vi "Two Force Sensors V3.vi"(8 "error out":errorcluster, 9 "Analog Input Pin 2":u8, 10 "Analog Input Pin1":u8, 11 "Arduino Resource":T1={"VISA resource"="", "Board Type"=enum."Uno", "Connection Type"=enum."USB / Serial", "Bytes Per Packet (15)"=15}) -> (0 "error out 2":errorcluster, 2 "Average Force":dbl(graph), 3 "Arduino Resource 2":T1={"VISA resource"="", "Board Type"=enum."Uno", "Connection Type"=enum."USB / Serial", "Bytes Per Packet (15)"=15})   [LabVIEW 2013]
uses:
  <vilib>/LabVIEW Interface for Arduino/Type Defs/Arduino Resource.ctl
  <vilib>/LabVIEW Interface for Arduino/Type Defs/Board Type.ctl
  <vilib>/Analysis/baseanly.llb/Mean (DBL).vi
  <vilib>/LabVIEW Interface for Arduino/LabVIEW Interface for Arduino.lvlib
  <vilib>/Analysis/NI_AALBase.lvlib
panel:
  out "Average Force":dbl
  out "Force2 Average":dbl format="%0.2f"
  out "Force1 Average":dbl format="%0.2f"
  out "Force 2":dbl(graph)
  out "Voltage2":dbl(graph)
  out "Force":dbl(graph)
  in  "Array":dbl[](array[numeric])
  in  "Stop":bool
  out "Volatge":dbl(graph)
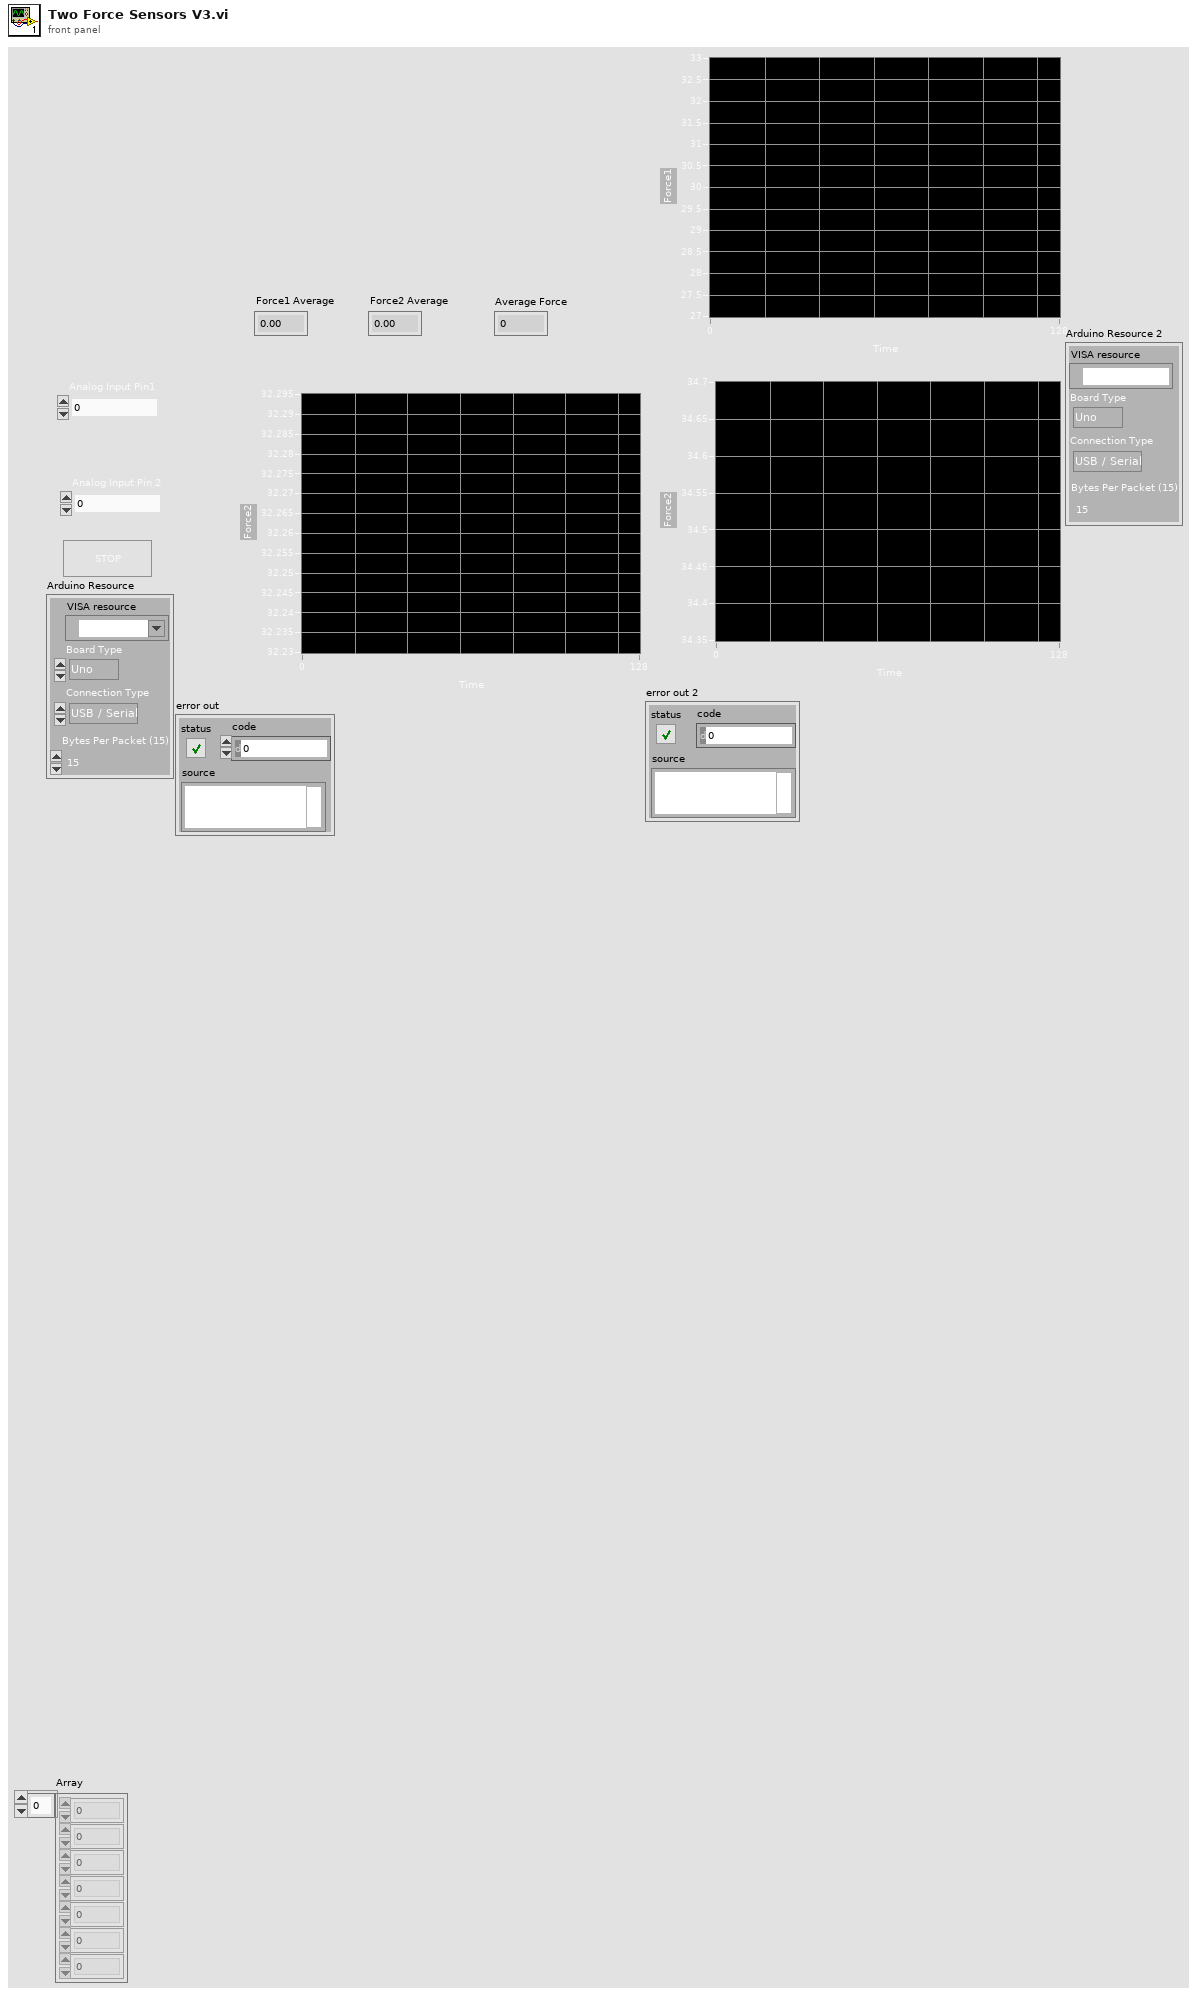
[diagram p1: front panel]
types:
  T1 = typedef "LabVIEW Interface for Arduino.lvlib/Arduino Resource.ctl" = cluster{"VISA resource":refnum<visa-resource-name>, "Board Type":T2, "Connection Type":enum8{"USB / Serial"}, "Bytes Per Packet (15)":u8}
  T2 = typedef "LabVIEW Interface for Arduino.lvlib/Board Type.ctl" = enum16{"Uno", "Dimuelanove w/Atmega 328", "Mega 2560"}
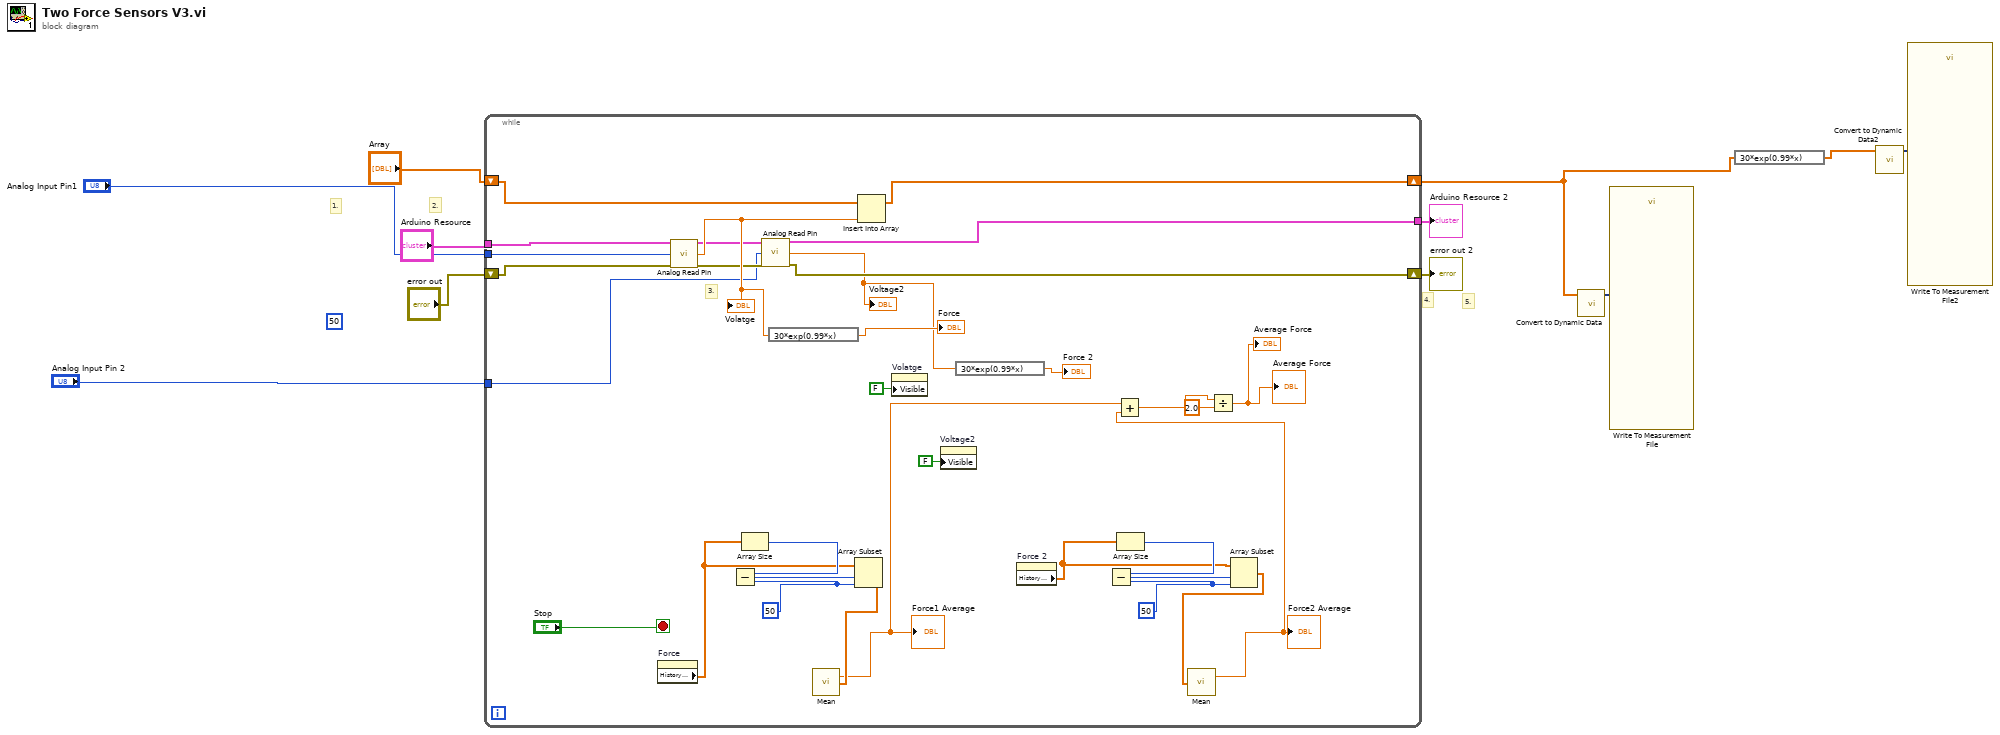
[diagram p0: block diagram]
diagram:
  (unwired) u16 50 ("Sample Rate (HZ)")
  # "5."
  # "4."
  # "2."
  # "1."
  n1 = while {
    shift-right: [w31] -> w1
    shift-left: "error out" -> [w12]
    shift-right: [w41] -> w9
    shift-left: "Array" -> [w42]
    tunnel: "Arduino Resource" -> [w36]
    tunnel: "Analog Input Pin1" -> [w35]
    tunnel: [w32] -> w2
    tunnel: "Analog Input Pin 2" -> [w14]
    stop <- "Stop" stop-if-true
    w22 = 50 ("length")
    w26 = 50 ("length")
    # "3."
    n2 = property on="Force" class="WFChart (strict)"() -> ("History Data"=w24:dbl[])  [unwired: 2 in, 2 out]
    n3 = call <vilib>:"Analog Read Pin.vi"("Arduino Resource"=w36, "Analog Input Pin (0)"=w35, "error in"=w12) -> ("Arduino Resource"=w34:T1, "Voltage"=w37:dbl, "error out"=w33:errorcluster)  [unwired: 10 in]
    "Volatge" <- w37
    n4 = Array Size(array=w24) -> (size(s)=w27:i32)
    n5 = Subtract(x=w27, y=w26) -> (x-y=w25:i32)
    n6 = call <vilib>:"Analog Read Pin.vi"("Arduino Resource"=w34, "Analog Input Pin (0)"=w14, "error in"=w33) -> ("Arduino Resource"=w32:T1, "Voltage"=w30:dbl, "error out"=w31:errorcluster)  [unwired: 10 in]
    "Voltage2" <- w30
    n7 = expression code="30*exp(0.99*x)"(w37) -> (→"Force":dbl)
    n8 = Array Subset(array=w24, index=w25, length=w26) -> (w28:dbl[])
    n9 = call-poly <vilib>:"Mean.vi"("X"=w28) -> ("mean"=w17:dbl)  [unwired: 1 out]
    "Force1 Average" <- w17
    n10 = Insert Into Array(array=w42, new element=w37) -> (w41:dbl[])  [unwired: 1 in]
    n11 = property on="Volatge" class="WFChart (strict)"("Visible"=FALSE) -> ()  [unwired: 2 in, 2 out]
    n12 = property on="Voltage2" class="WFChart (strict)"("Visible"=FALSE) -> ()  [unwired: 2 in, 2 out]
    n13 = expression code="30*exp(0.99*x)"(w30) -> (→"Force 2":dbl)
    n14 = property on="Force 2" class="WFChart (strict)"() -> ("History Data"=w20:dbl[])  [unwired: 2 in, 2 out]
    n15 = Array Size(array=w20) -> (size(s)=w23:i32)
    n16 = Subtract(x=w23, y=w22) -> (x-y=w21:i32)
    n17 = Array Subset(array=w20, index=w21, length=w22) -> (w19:dbl[])
    n18 = call-poly <vilib>:"Mean.vi"("X"=w19) -> ("mean"=w16:dbl)  [unwired: 1 out]
    "Force2 Average" <- w16
    n19 = Add(x=w17, y=w16) -> (x+y=w15:dbl)
    n20 = Divide(x=w15, y=2.0) -> (x/y=→"Average Force" →"Average Force":dbl)
  }
  "Arduino Resource 2" <- w2
  "error out 2" <- w1
  n21 = call "Convert to Dynamic Data"("Array"=w9) -> ("Dynamic Data Type"=w10:dynamicdata)  [unwired: 3 in]
  n22 = call "Write To Measurement File"("Signals"=w10) -> ()  [unwired: 16 in, 3 out]
  n23 = expression code="30*exp(0.99*x)"(w9) -> (w8:dbl[])
  n24 = call "Convert to Dynamic Data2"("Array"=w8) -> ("Dynamic Data Type"=w7:dynamicdata)  [unwired: 3 in]
  n25 = call "Write To Measurement File2"("Signals"=w7) -> ()  [unwired: 16 in, 3 out]
